vi "pi_scan.vi"(8 "error in":errorcluster, 10 "Start Position":dbl=9.0) -> (0 "error out":errorcluster, 2 "Current position":dbl)   [LabVIEW 2014]
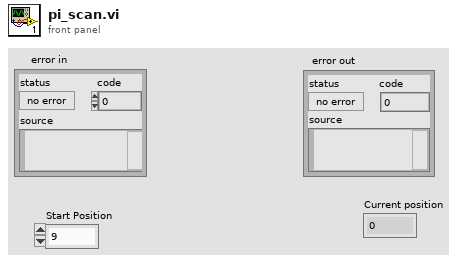
[diagram p1: front panel]
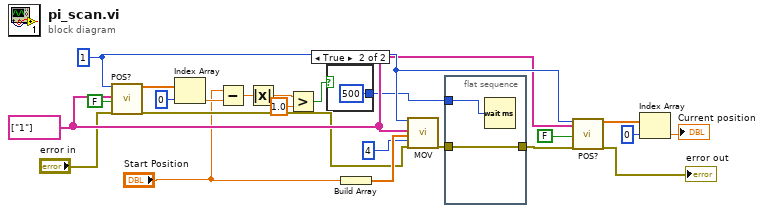
[diagram p0: block diagram]
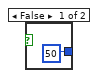
[diagram p2: hidden frame]
diagram:
  w15 = 1 ("System no.")
  w14 = string[] ["1"] ("Axes to move")
  n1 = call "POS?.vi"("System no."=w15, "Axes to query"=w14, "All axes?"=FALSE, "error in"="error in") -> ("Position"=w11:dbl[], "error out"=w13:errorcluster)  [unwired: 14 in]
  n2 = Index Array(array=w11, index=0) -> (element=w9:dbl)
  n3 = Subtract(x="Start Position", y=w9) -> (x-y=w8:dbl)
  n4 = Absolute Value(x=w8) -> (abs(x)=w7:dbl)
  n5 = Greater?(x=w7, y=1.0) -> (0:w5:bool)
  n6 = case shown="True" w5 {
    tunnel: [u32 50 ("milliseconds to wait") u32 500 ("milliseconds to wait")] -> w4
    frame False {
    }
    frame True {
    }
  }
  n7 = Build Array("Start Position") -> (w23:dbl[])
  n8 = call "MOV.vi"("System no."=w15, "Axes to move"=w14, "Position values"=w23, "No.of digits"=i16 4, "error in"=w13) -> ("error out"=w17:errorcluster)  [unwired: 14 in]
  n9 = flat-sequence {
    tunnel: w17 -> [w27]
    tunnel: [w27] -> w16
    tunnel: w4 -> [w26]
    frame #0 {
      n10 = Wait (ms)(milliseconds to wait=w26) -> ()  [unwired: 1 out]
    }
  }
  n11 = call "POS?.vi"("System no."=w15, "Axes to query"=w14, "All axes?"=FALSE, "error in"=w16) -> ("Position"=w20:dbl[], "error out"=→"error out":errorcluster)  [unwired: 14 in]
  n12 = Index Array(array=w20, index=0) -> (element=→"Current position":dbl)
